vi "cv_04-05_dice.vi"() -> ()   [LabVIEW 2013]
panel:
  out "Index Array":u8[](array[numeric])
  out "XY Graph":cluster{i32[], i32[]}(graph)
  out "Histogram":u8[](array[numeric])
  out "Array":u8[](array[numeric])
  in  "# to roll die":u16
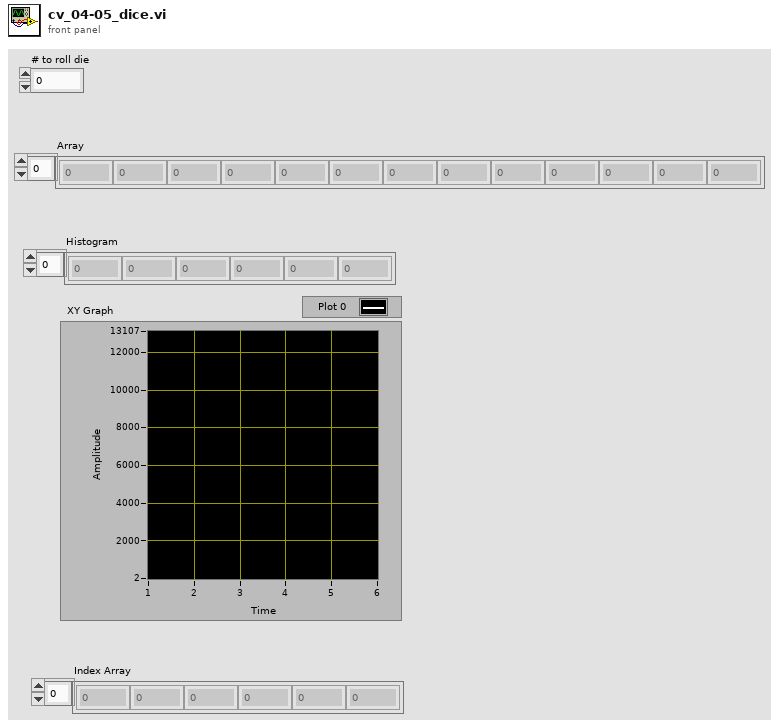
[diagram p1: front panel]
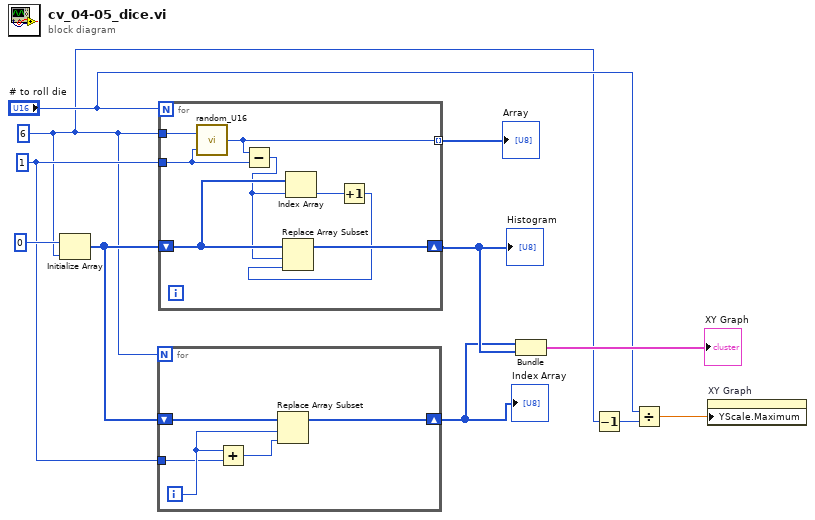
[diagram p0: block diagram]
diagram:
  w2 = 1
  w1 = 6
  n1 = Initialize Array(0, w1) -> (w8:i32[])
  n2 = for {
    N: w1 -> [_]
    shift-right: [w15] -> w7
    shift-left: w8 -> [w16]
    tunnel: w2 -> [w12]
    i -> [w13]
    n3 = Add(x=w13, y=w12) -> (x+y=w14:i32)
    n4 = Replace Array Subset(array=w16, new element=w14, index=w13) -> (w15:i32[])
  }
  "Index Array" <- w7
  n5 = for {
    N: "# to roll die" -> [_]
    tunnel: [w21] -> w11 mode=indexing
    tunnel: w1 -> [w24]
    shift-right: [w20] -> w9
    shift-left: w8 -> [w23]
    tunnel: w2 -> [w17]
    n6 = call "random_U16.vi"("Offset"=w17, "Range"=w24) -> ("Out"=w21:u16)
    n7 = Subtract(x=w21, y=w17) -> (x-y=w18:i32)
    n8 = Index Array(array=w23, index=w18) -> (element=w22:i32)
    n9 = Increment(x=w22) -> (x+1=w19:i32)
    n10 = Replace Array Subset(array=w23, new element=w19, index=w18) -> (w20:i32[])
  }
  "Array" <- w11
  "Histogram" <- w9
  n11 = Bundle(w7, w9) -> (→"XY Graph":cluster{i32[], i32[]})  [unwired: 1 in]
  n12 = Decrement(x=w1) -> (x-1=w3:i32)
  n13 = Divide(x="# to roll die", y=w3) -> (x/y=w5:dbl)
  n14 = property on="XY Graph" class="XYGraph (strict)"("YScale.Maximum"=w5) -> ()  [unwired: 2 in, 2 out]
